vi "Get Filtered Base System Images.vi"(5 "Device Class":string, 6 "Product ID":i32 format="%.0x", 7 "Operating System":string, 8 "error in (no error)":errorcluster, 11 "Repository in (RT Images)":path) -> (0 "error out":errorcluster, 2 "Base System Images":T1[](array[typedef]) {"component type" items=["standard", "hidden", "system", "unknown", "startup", "image", "essential"]}, 3 "Repository out":path)   [LabVIEW 2017, in "nisyscfg.lvlib"]
doc: "Retrieves a collection of base system images available from a repository path."
uses:
  <vilib>/nisyscfg/nisyscfg.lvlib
  <vilib>/nisyscfg/Software 1.2.ctl
  <vilib>/nisyscfg/Component Type.ctl
  <resource>/objmgr/nisysapi.rc
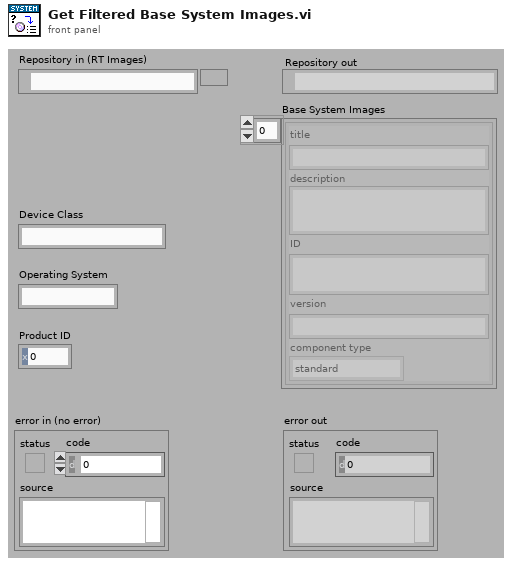
[diagram p1: front panel]
types:
  T1 = typedef "nisyscfg.lvlib/Software 1.2.ctl" = cluster{"title":string, "description":string, "ID":string, "version":string, "component type":T2}
  T2 = typedef "nisyscfg.lvlib/Component Type.ctl" = u32
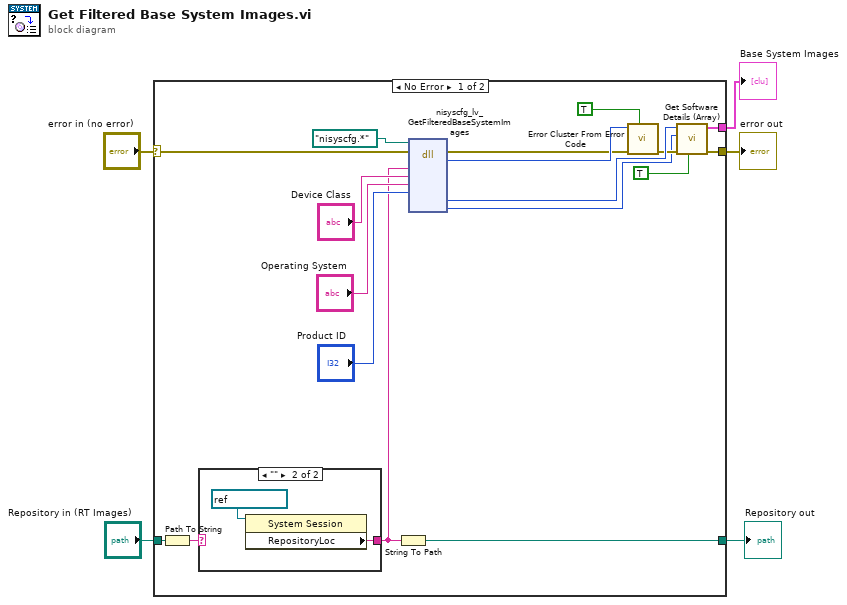
[diagram p0: block diagram]
diagram:
  n1 = case shown="No Error" "error in (no error)" {
    selector: "error in (no error)" -> [w21 w28]
    tunnel: [w16 w28] -> w5
    tunnel: "Repository in (RT Images)" -> [w9 w27]
    tunnel: [w15 _] -> w2
    tunnel: [w6 w27] -> w1
    frame No Error {
      n2 = Path To String(path=w9) -> (string=w8:string)
      n3 = case shown="\"\"" w8 {
        selector: w8 -> [w24 _]
        tunnel: [w24 w26] -> w7
        frame Default {
        }
        frame "" {
          n4 = property class="System Session"(reference=refnum<k21> "localhost" ("System Configuration")) -> ("RepositoryLoc"=w26:string)  [unwired: 1 in, 2 out]
        }
      }
      n5 = String To Path(string=w7) -> (path=w6:path)
      n6 = dll-call lib="nisyscfg.*" fn="nisyscfg_lv_GetFilteredBaseSystemImages" label="GetFilteredBaseSystemImages"(path in=path "nisyscfg.*", error in=w21, "repository"=w7, "deviceClass"="Device Class", "operatingSystem"="Operating System", "productID"="Product ID") -> (error out=w22:errorcluster, "result"=w23:i32, "systemImages"=w18:u64, "numSystemImages"=w14:i32)  [unwired: 7 in, 1 out]
      n7 = call <vilib>:"Error Cluster From Error Code.vi"("show call chain? (False)"=TRUE, "error in (no error)"=w22, "error code (0)"=w23) -> ("error out"=w17:errorcluster)  [unwired: 6 in]
      n8 = call <vilib>:"Get Software Details (Array).vi"("Trace Component Info (F)"=TRUE ("log to NI Spy (F)"), "error in (no error)"=w17, "Number of Elements"=w14, "Enumerator in"=w18) -> ("error out"=w16:errorcluster, "Software Components"=w15:T1[])  [unwired: 6 in]
    }
    frame Error {
    }
  }
  "error out" <- w5
  "Base System Images" <- w2
  "Repository out" <- w1
